vi "sub_SDR_siso_AddPilots.vi"(10 "Array in":cdb[](array[numeric]), 11 "Symbols/Pilots":i32) -> (2 "Array Out":cdb[](array[numeric]))   [LabVIEW 2012]
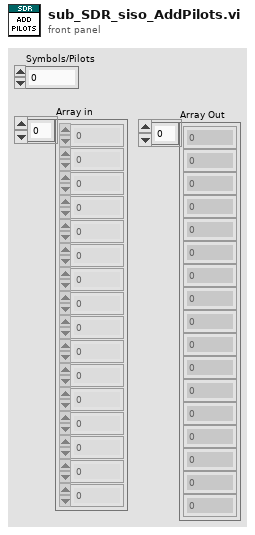
[diagram p1: front panel]
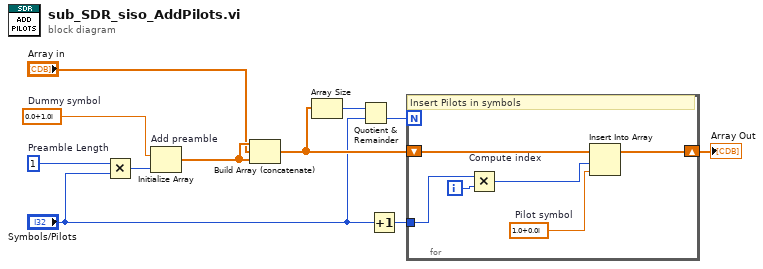
[diagram p0: block diagram]
diagram:
  w1 = 1  # Preamble Length
  w5 = cdb 0.0+1.0i  # Dummy symbol
  n1 = Multiply(x=w1, y="Symbols/Pilots") -> (x*y=w3:i32)
  n2 = Initialize Array "Add preamble"(w5, w3) -> (w11:cdb[])
  n3 = Build Array (concatenate) "Build Array"(w11, "Array in", w11) -> (w7:cdb[])
  n4 = Array Size(array=w7) -> (size(s)=w9:i32)
  n5 = Quotient & Remainder(x=w9, y="Symbols/Pilots") -> (floor(x/y)=w8:i32)  [unwired: 1 out]
  n6 = Increment(x="Symbols/Pilots") -> (x+1=w4:i32)
  n7 = for {
    N: w8 -> [_]
    tunnel: w4 -> [w16]
    shift-right: [w14] -> w10
    shift-left: w7 -> [w17]
    i -> [w13]
    w12 = cdb 1.0+0.0i  # Pilot symbol
    # "Insert Pilots in symbols"
    n8 = Multiply "Compute index"(x=w16, y=w13) -> (x*y=w15:i32)
    n9 = Insert Into Array "Insert Into Array"(array=w17, index=w15, new element=w12) -> (w14:cdb[])
  }
  "Array Out" <- w10
